vi "Initialize.vi"(7 "Components":refnum<class "Component.lvclass">[](array[class]), 8 "error in (no error)":errorcluster, 10 "Plugin Configuration":refnum<class "Plugin Configuration.lvclass">, 11 "Transceiver Thread in":refnum<class "Transceiver Thread.lvclass">) -> (0 "error out":errorcluster, 3 "Transceiver Thread out":refnum<class "Transceiver Thread.lvclass">)   [LabVIEW 2017, in "DSF Core.lvlib" / "Transceiver Thread.lvclass"]
uses:
  Transceiver Thread.lvclass
  C:/Git/DSF/Core/Classes/Thread/Thread.lvclass
  Component/Component.lvclass
  Configuration/Core/Plugin/Plugin Configuration.lvclass
  Configuration/Core/Plugin/Plugin Configuration.lvclass/Plugin Configuration.ctl
  Configuration/Core/Thread/Thread Configuration.lvclass/Thread Configuration.ctl
  Configuration/Core/Core Configuration.lvclass/Core Configuration.ctl
  Transceiver Thread.lvclass/Transceiver Thread.ctl
  Configuration/Core/Thread/Thread Configuration.lvclass
  C:/Git/DSF/Core/Classes/Configuration/Core/Core Configuration.lvclass
  Buffer Converter/Buffer Converter.lvclass
  Transceiver/Transceiver.lvclass
  Configuration/Core/Core Configuration.lvclass
  Thread.lvclass
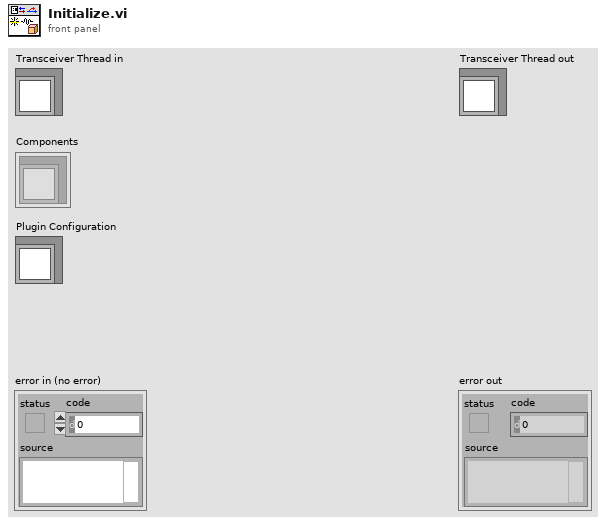
[diagram p1: front panel]
types:
  T1 = typedef "DSF Core.lvlib/DSF Settings Info.ctl" = cluster{"component":string, "values":cluster{"key":string, "value":string}[]}
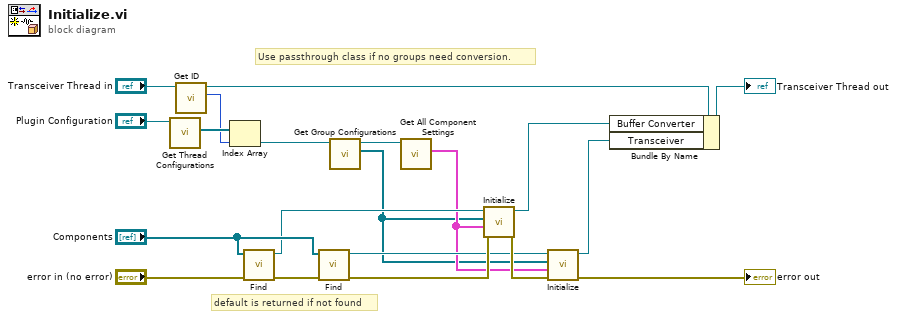
[diagram p0: block diagram]
diagram:
  # "Use passthrough class if no groups need conversion."
  # "default is returned if not found"
  n1 = call "Get Thread Configurations.vi"("Plugin Configuration in"="Plugin Configuration") -> ("Thread Configurations"=w3:refnum<class "Thread Configuration.lvclass">[])  [unwired: 8 in, 2 out]
  n2 = call "Get ID.vi"("Thread in"="Transceiver Thread in") -> ("ID"=w2:i32, "Thread out"=w5:refnum<class "Transceiver Thread.lvclass">)  [unwired: 9 in]
  n3 = Index Array(array=w3, index=w2) -> (element=w1:refnum<class "Thread Configuration.lvclass">)
  n4 = call "Find.vi"("error in (no error)"="error in (no error)", "Components"="Components") -> ("error out"=w20:errorcluster, "Buffer Converter"=w10:refnum<class "Buffer Converter.lvclass">)  [unwired: 7 in, 1 out]
  n5 = call "Find.vi"("error in (no error)"=w20, "Components"="Components") -> ("error out"=w15:errorcluster, "Transceiver"=w11:refnum<class "Transceiver.lvclass">)  [unwired: 7 in, 1 out]
  n6 = call "Get Group Configurations.vi"("Thread Configuration in"=w1) -> ("Group Configurations"=w7:refnum<class "Group Configuration.lvclass">[], "Thread Configuration out"=w8:refnum<class "Thread Configuration.lvclass">)  [unwired: 8 in, 1 out]
  n7 = call "Get All Component Settings.vi"("Runtime Configuration in"=w8) -> ("component settings"=w9:T1[])  [unwired: 8 in, 2 out]
  n8 = call-dynamic "Initialize.vi"("error in (no error)"=w15, "thread settings"=w9, "Group Configurations"=w7, "Buffer Converter in"=w10) -> ("error out"=w16:errorcluster, "Buffer Converter out"=w13:refnum<class "Buffer Converter.lvclass">)  [unwired: 6 in]
  n9 = call-dynamic "Initialize.vi"("error in (no error)"=w16, "thread settings"=w9, "Group Configurations"=w7, "Transceiver in"=w11) -> ("error out"=→"error out":errorcluster, "Transceiver out"=w12:refnum<class "Transceiver.lvclass">)  [unwired: 6 in]
  n10 = Bundle By Name(cluster=w5, "Buffer Converter"=w13, "Transceiver"=w12) -> (→"Transceiver Thread out":refnum<class "Transceiver Thread.lvclass">)
